vi "profile.vi"(1 "Input Parameters Cluster":T1={"nu0"=112265.5949, "GammaD"=0.0351, "Gamma0"=0.0117, "Gamma2"=0.0054, "Delta0"=0.0305, "Delta2"=0.0124, "NuOptRe"=0.038, "NuOptIm"=-0.0175, "nu"=112266.5949, "Xlm"=0.001, "Ylm"=0.0005, "alpha"=1.98573285442, "disp"=enum."Absorption"} {"alpha" format="%#_16f"; "Ylm" format="%#_16f"; "Xlm" format="%#_16f"; "nu0" format="%#_16g"; "GammaD" format="%#_16f"; "Gamma0" format="%#_16f"; "Gamma2" format="%#_16f"; "Delta0" format="%#_16f"; "Delta2" format="%#_16f"; "NuOptRe" format="%#_16f"; "NuOptIm" format="%#_16f"; "nu" format="%#_16f"}) -> (0 "mHT":dbl=0.004070823872413185 format="%#_16g")   [LabVIEW 2015]
panel:
  out "nu'":cdb=0.03283813126429161-1.0056i format="%#_13g"
  in  "rp":dbl=1.772453850905516 format="%#_13g"
  in  "numinf":dbl=4000.0 format="%#_13g"
  in  "num0":dbl=1e-15 format="%#_13g"
  out "c0":cdb=0.03283813126429161-0.005600000000000001i format="%#_13g"
  out "c2":cdb=0.0054+0.0124i format="%#_13g"
  out "nuD":cdb=0.04215939654840439+0.0i format="%#_13g"
  # "modified Hartman Tran profile"
  # "Subroutine to compute the complex normalized spectral-line shape using mHT model\n\nStandard Input Parameters:\n--------------------\nnu0     : Unperturbed line position in cm-1.\nGammaD  : Doppler broadening in cm-1.\nGamma0  : Speed-averaged line-width in cm-1.       \nGamma2  : Quadratic speed dependence parameter of the line-width in cm-1.\nDelta0  : Speed-averaged line-shift in cm-1.\nDelta2  : Quadratic speed dependence parameter of the line-shift in cm-1.   \nNuOptRe : Real part of the complex Dicke parameter in cm-1.\nNuOptIm : Imaginary part of the complex Dicke parameter in cm-1.    \nnu      : Current WaveNumber in cm-1.\nYlm     : Imaginary part of the 1st order (Rosenkranz) line mixing \n          coefficients, dimensionless (default: 0.0).\nXlm     : Real part of the 1st order (Rosenkranz) line mixing \n          coefficients, dimensionless (default: 0.0).\nalpha   : Mass ratio in the molecule for calculating beta-correction, \n          applicable up to alpha=5, dimensionless (default: 10.0).\ndisp    : Boolean trigger for including dispersion profile \n          in the output (default: Absorption).\n\nThe function has one outputs:\n--------------------\n(1)     : Real or imaginary (depending on disp value) part of the \n          normalized spectral shape in cm."
  # "Input Section"
  # "Output Section"
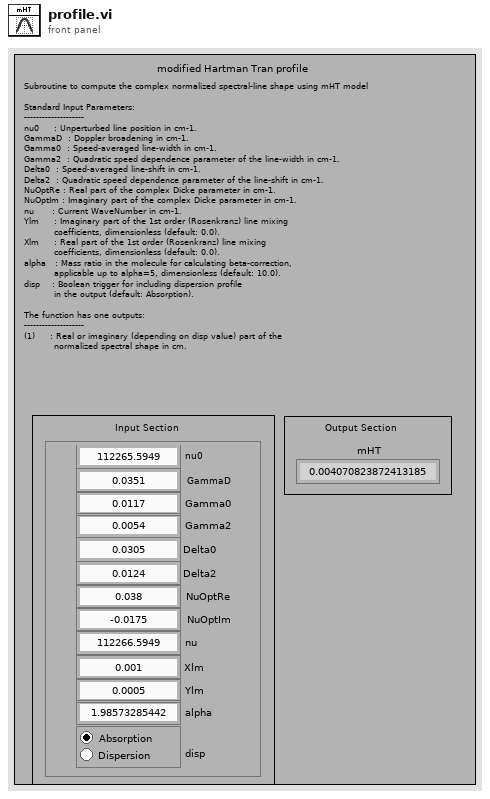
[diagram p1: front panel]
types:
  T1 = cluster{"nu0":dbl, "GammaD":dbl, "Gamma0":dbl, "Gamma2":dbl, "Delta0":dbl, "Delta2":dbl, "NuOptRe":dbl, "NuOptIm":dbl, "nu":dbl, "Xlm":dbl, "Ylm":dbl, "alpha":dbl, "disp":enum32{"Absorption", "Dispersion"}}
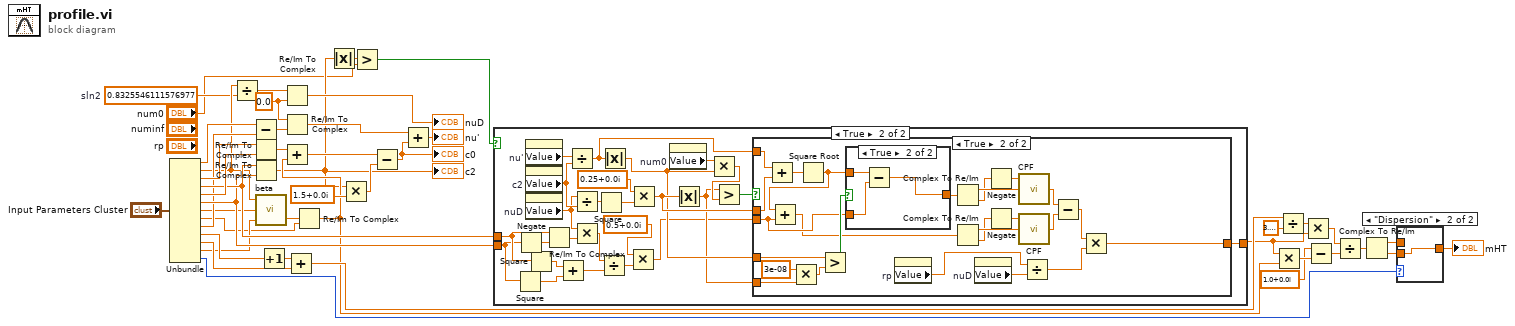
[diagram p0: block diagram]
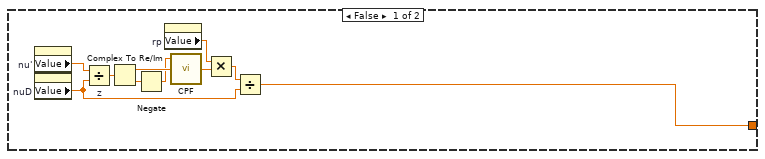
[diagram p3: hidden frame]
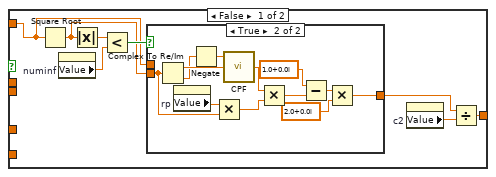
[diagram p4: hidden frame]
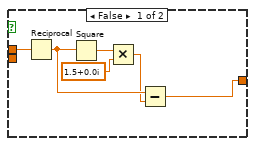
[diagram p5: hidden frame]
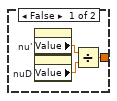
[diagram p6: hidden frame]
diagram:
  w25 = 0.0 ("x")
  w9 = 0.8325546111576977  # sln2
  n1 = Unbundle("Input Parameters Cluster") -> ("nu0"=w41:dbl, "GammaD"=w15:dbl, "Gamma0"=w43:dbl, "Gamma2"=w40:dbl, "Delta0"=w42:dbl, "Delta2"=w39:dbl, "NuOptRe"=w14:dbl, "NuOptIm"=w8:dbl, "nu"=w38:dbl, "Xlm"=w17:dbl, "Ylm"=w16:dbl, "alpha"=w13:dbl, "disp"=w6:enum32{"Absorption", "Dispersion"})
  n2 = Divide(x=w15, y=w9) -> (x/y=w24:dbl)
  n3 = Subtract(x=w41, y=w38) -> (x-y=w37:dbl)
  n4 = Re/Im To Complex(1:w42, 2:w43) -> (0:w36:cdb)
  n5 = Re/Im To Complex(1:w39, 2:w40) -> (0:w4:cdb)
  "c2" <- w4
  n6 = call "beta.vi"("alpha"=w13, "NuOptRe"=w14, "GammaD"=w15) -> ("nuR"=w12:dbl)  [unwired: 1 out]
  n7 = Increment(x=w17) -> (x+1=w18:dbl)
  n8 = Re/Im To Complex(1:w25, 2:w24) -> (0:→"nuD":cdb)
  n9 = Re/Im To Complex(1:w37, 2:w25) -> (0:w35:cdb)
  n10 = Add(x=w18, y=w16) -> (x+y=w7:dbl)
  n11 = Re/Im To Complex(1:w8, 2:w12) -> (0:w5:cdb)
  n12 = Add(x=w36, y=w5) -> (x+y=w26:cdb)
  n13 = Absolute Value(x=w4) -> (abs(x)=w44:dbl)
  n14 = Multiply(x=w4, y=cdb 1.5+0.0i ("x")) -> (x*y=w10:cdb)
  n15 = Greater?(x=w44, y="num0") -> (0:w32:bool)
  n16 = Subtract(x=w26, y=w10) -> (x-y=w34:cdb)
  "c0" <- w34
  n17 = Add(x=w35, y=w34) -> (x+y=→"nu'":cdb)
  n18 = case shown="True" w32 {
    tunnel: w40 -> [_ w74]
    tunnel: w39 -> [_ w56]
    tunnel: [w49 w57] -> w2
    frame False {
      n19 = property on="nu'" class="DigNum (strict)"() -> ("Value"=w48:cdb)  [unwired: 2 in, 2 out]
      n20 = property on="nuD" class="DigNum (strict)"() -> ("Value"=w47:cdb)  [unwired: 2 in, 2 out]
      n21 = Divide "z"(x=w48, y=w47) -> (x/y=w55:cdb)
      n22 = Complex To Re/Im(x + iy=w55) -> (x=w53:dbl, y=w54:dbl)
      n23 = Negate(x=w54) -> (-x=w52:dbl)
      n24 = property on="rp" class="DigNum (strict)"() -> ("Value"=w46:dbl)  [unwired: 2 in, 2 out]
      n25 = call "CPF.vi"("y"=w53, "x"=w52) -> ("CPF"=w51:cdb)  [unwired: 1 in]
      n26 = Multiply(x=w46, y=w51) -> (x*y=w50:cdb)
      n27 = Divide(x=w50, y=w47) -> (x/y=w49:cdb)
    }
    frame True {
      n28 = Square(x=w56) -> (x^2=w72:dbl)
      n29 = Negate(x=w56) -> (-x=w75:dbl)
      n30 = property on="nu'" class="DigNum (strict)"() -> ("Value"=w80:cdb)  [unwired: 2 in, 2 out]
      n31 = property on="c2" class="DigNum (strict)"() -> ("Value"=w79:cdb)  [unwired: 2 in, 2 out]
      n32 = property on="nuD" class="DigNum (strict)"() -> ("Value"=w70:cdb)  [unwired: 2 in, 2 out]
      n33 = Square(x=w74) -> (x^2=w73:dbl)
      n34 = Re/Im To Complex(1:w75, 2:w74) -> (0:w71:cdb)
      n35 = Add(x=w73, y=w72) -> (x+y=w69:dbl)
      n36 = Divide(x=w80, y=w79) -> (x/y=w62:cdb)
      n37 = Divide(x=w70, y=w79) -> (x/y=w78:cdb)
      n38 = Multiply(x=w70, y=w71) -> (x*y=w68:cdb)
      n39 = Square(x=w78) -> (x^2=w77:cdb)
      n40 = Divide(x=w68, y=w69) -> (x/y=w67:cdb)
      n41 = Absolute Value(x=w62) -> (abs(x)=w60:dbl)
      n42 = Multiply(x=cdb 0.5+0.0i, y=w67) -> (x*y=w58:cdb)
      n43 = Multiply(x=cdb 0.25+0.0i, y=w77) -> (x*y=w61:cdb)
      n44 = property on="num0" class="DigNum (strict)"() -> ("Value"=w65:dbl)  [unwired: 2 in, 2 out]
      n45 = Absolute Value(x=w61) -> (abs(x)=w59:dbl)
      n46 = Multiply(x=w65, y=w60) -> (x*y=w64:dbl)
      n47 = Greater?(x=w59, y=w64) -> (0:w63:bool)
      n48 = case shown="True" w63 {
        tunnel: w62 -> [w81 w129]
        tunnel: w61 -> [_ w131]
        tunnel: w60 -> [_ w125]
        tunnel: w59 -> [_ w128]
        tunnel: w58 -> [_ w122]
        tunnel: [w82 w107] -> w57
        frame False {
          n49 = Square Root(x=w81) -> (sqrt(x)=w85:cdb)
          n50 = property on="numinf" class="DigNum (strict)"() -> ("Value"=w87:dbl)  [unwired: 2 in, 2 out]
          n51 = Absolute Value(x=w85) -> (abs(x)=w88:dbl)
          n52 = Less?(x=w88, y=w87) -> (x < y?=w86:bool)
          n53 = case shown="True" w86 {
            tunnel: w85 -> [_ w102]
            tunnel: [w89 w95] -> w83
            tunnel: w81 -> [w94 _]
            frame False {
              n54 = Reciprocal(x=w94) -> (1/x=w91:cdb)
              n55 = Square(x=w91) -> (x^2=w93:cdb)
              n56 = Multiply(x=w93, y=cdb 1.5+0.0i) -> (x*y=w90:cdb)
              n57 = Subtract(x=w91, y=w90) -> (x-y=w89:cdb)
            }
            frame True {
              n58 = Complex To Re/Im(x + iy=w102) -> (x=w106:dbl, y=w104:dbl)
              n59 = property on="rp" class="DigNum (strict)"() -> ("Value"=w103:dbl)  [unwired: 2 in, 2 out]
              n60 = Negate(x=w104) -> (-x=w105:dbl)
              n61 = Multiply(x=w103, y=w102) -> (x*y=w101:cdb)
              n62 = call "CPF.vi"("y"=w106, "x"=w105) -> ("CPF"=w100:cdb)  [unwired: 1 in]
              n63 = Multiply(x=w100, y=w101) -> (x*y=w99:cdb)
              n64 = Subtract(x=cdb 1.0+0.0i, y=w99) -> (x-y=w97:cdb)
              n65 = Multiply(x=w97, y=cdb 2.0+0.0i) -> (x*y=w95:cdb)
            }
          }
          n66 = property on="c2" class="DigNum (strict)"() -> ("Value"=w84:cdb)  [unwired: 2 in, 2 out]
          n67 = Divide(x=w83, y=w84) -> (x/y=w82:cdb)
        }
        frame True {
          n68 = Add(x=w129, y=w131) -> (x+y=w130:cdb)
          n69 = Multiply(x=3e-08, y=w128) -> (x*y=w126:dbl)
          n70 = Square Root(x=w130) -> (sqrt(x)=w123:cdb)
          n71 = Add(x=w123, y=w122) -> (x+y=w114:cdb)
          n72 = Greater?(x=w125, y=w126) -> (0:w124:bool)
          n73 = case shown="True" w124 {
            tunnel: w123 -> [_ w137]
            tunnel: w122 -> [_ w136]
            tunnel: [w132 w135] -> w121
            frame False {
              n74 = property on="nu'" class="DigNum (strict)"() -> ("Value"=w134:cdb)  [unwired: 2 in, 2 out]
              n75 = property on="nuD" class="DigNum (strict)"() -> ("Value"=w133:cdb)  [unwired: 2 in, 2 out]
              n76 = Divide(x=w134, y=w133) -> (x/y=w132:cdb)
            }
            frame True {
              n77 = Subtract(x=w137, y=w136) -> (x-y=w135:cdb)
            }
          }
          n78 = property on="rp" class="DigNum (strict)"() -> ("Value"=w110:dbl)  [unwired: 2 in, 2 out]
          n79 = Complex To Re/Im(x + iy=w121) -> (x=w120:dbl, y=w118:dbl)
          n80 = Complex To Re/Im(x + iy=w114) -> (x=w117:dbl, y=w115:dbl)
          n81 = property on="nuD" class="DigNum (strict)"() -> ("Value"=w111:cdb)  [unwired: 2 in, 2 out]
          n82 = Negate(x=w118) -> (-x=w119:dbl)
          n83 = Negate(x=w115) -> (-x=w116:dbl)
          n84 = call "CPF.vi"("y"=w120, "x"=w119) -> ("CPF"=w113:cdb)  [unwired: 1 in]
          n85 = call "CPF.vi"("y"=w117, "x"=w116) -> ("CPF"=w112:cdb)  [unwired: 1 in]
          n86 = Divide(x=w110, y=w111) -> (x/y=w108:cdb)
          n87 = Subtract(x=w113, y=w112) -> (x-y=w109:cdb)
          n88 = Multiply(x=w109, y=w108) -> (x*y=w107:cdb)
        }
      }
    }
  }
  n89 = Multiply(x=w2, y=w5) -> (x*y=w29:cdb)
  n90 = Divide(x=w7, y=3.141592653589793) -> (x/y=w30:dbl)
  n91 = Multiply(x=w30, y=w2) -> (x*y=w1:cdb)
  n92 = Subtract(x=cdb 1.0+0.0i, y=w29) -> (x-y=w27:cdb)
  n93 = Divide(x=w1, y=w27) -> (x/y=w22:cdb)
  n94 = Complex To Re/Im(x + iy=w22) -> (x=w21:dbl, y=w20:dbl)
  n95 = case shown="\"Dispersion\"" w6 {
    tunnel: w21 -> [w138 _]
    tunnel: w20 -> [_ w139]
    tunnel: [w138 w139] -> w19
    frame "Absorption", Default {
    }
    frame "Dispersion" {
    }
  }
  "mHT" <- w19
